vi "updateCommandString.vi"(8 "error in (no error)":errorcluster, 10 "Command U8 Array":u8[](array[numeric]), 11 "MiddlewareSALThisComponent in":refnum<class "MiddlewareSALThisComponent.lvclass">) -> (0 "error out":errorcluster, 2 "Cmd str":string, 3 "MiddlewareSALThisComponent out":refnum<class "MiddlewareSALThisComponent.lvclass">)   [LabVIEW 2016, in "MiddlewareSALThisComponent.lvclass"]
uses:
  MiddlewareSALThisComponent.lvclass
  ComponentTemplateCore/ComponentModel/ComponentModel/Command/Command.lvclass
  SALCommunicatorDL/SALCommunicatorDL.lvclass
  Commands/Start/Start.lvclass
  home/andres/ct_cmpuserevents/CommandThisComponent/CommandThisComponent.lvclass
  home/andres/ct_cmpuserevents/ComponentTemplateCore/ComponentModel/ComponentModel/Command/Command.lvclass
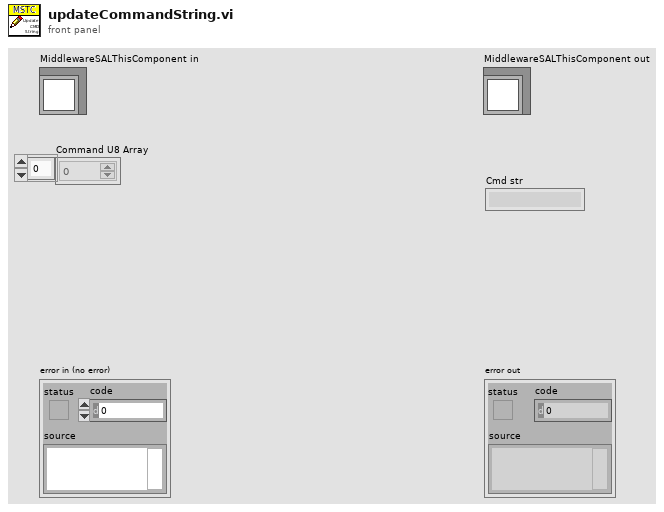
[diagram p1: front panel]
types:
  T1 = enum16{"Command", "Start", "ClearError", "HeartBeat", "Enable", "Disable", "Standby", "Exit", "OnInterrupt", "OnIncomingMessagingError"}
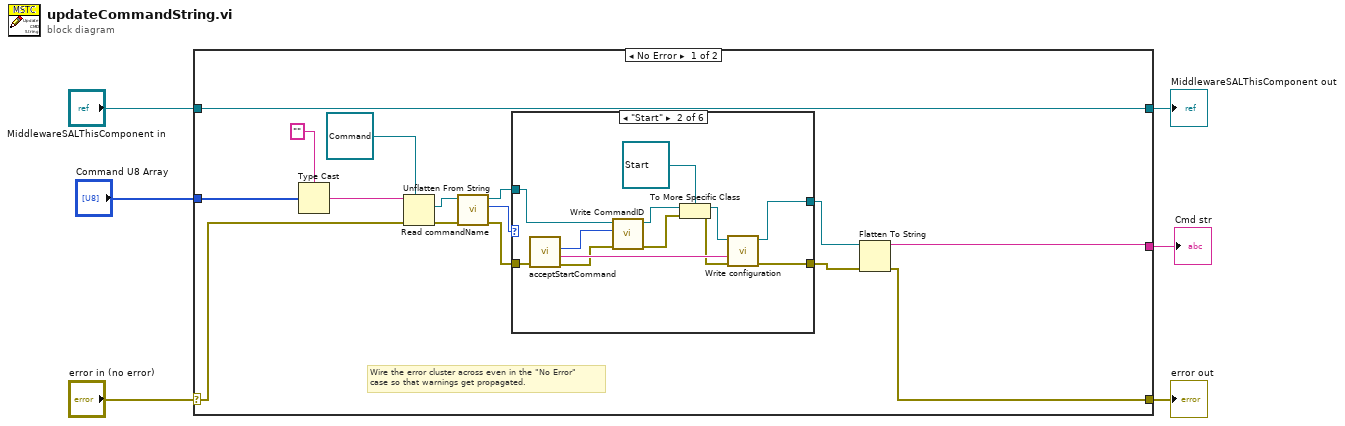
[diagram p0: block diagram]
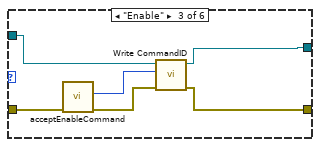
[diagram p3: hidden frame]
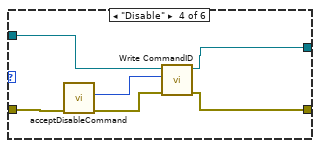
[diagram p4: hidden frame]
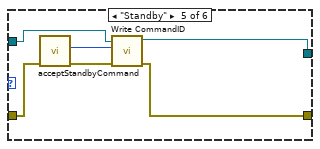
[diagram p5: hidden frame]
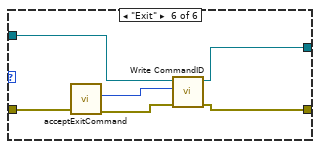
[diagram p6: hidden frame]
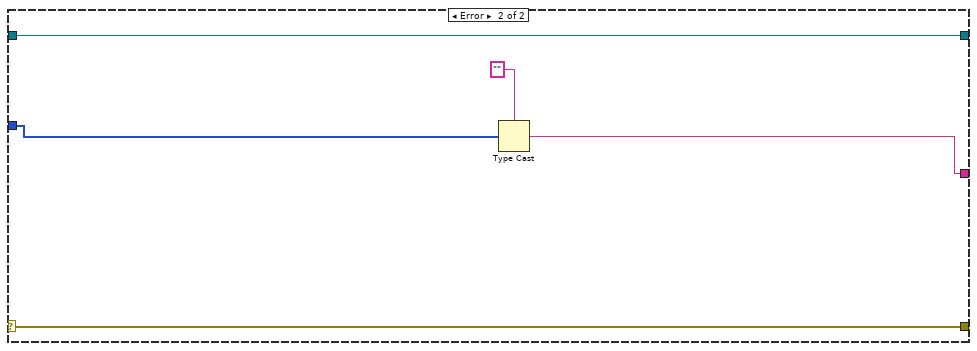
[diagram p7: hidden frame]
diagram:
  n1 = case shown="No Error" "error in (no error)" {
    selector: "error in (no error)" -> [w16 w64]
    tunnel: [w9 w64] -> w5
    tunnel: [w21 w63] -> w3
    tunnel: "MiddlewareSALThisComponent in" -> [w21 w63]
    tunnel: "Command U8 Array" -> [w17 w62]
    tunnel: [w7 w60] -> w1
    frame No Error {
      # "Wire the error cluster across even in the \"No Error\"\ncase so that warnings get propagated."
      n2 = Type Cast(type="", x=w17) -> (*(type *) &x=w18:string)
      n3 = Unflatten From String(type=refnum<class "Command.lvclass"> refnum ("Command.lvclass"), binary string=w18, error in (no error)=w16) -> (value=w14:refnum<class "Command.lvclass">, error out=w15:errorcluster)  [unwired: 2 in, 1 out]
      n4 = call-dynamic "Read commandName.vi"("error in (no error)"=w15, "Command in"=w14) -> ("error out"=w12:errorcluster, "Enum"=w13:T1, "Command out"=w11:refnum<class "Command.lvclass">)  [unwired: 7 in]
      n5 = case shown="\"Start\"" w13 {
        tunnel: w12 -> [w23 w35 w37 w46 w51 w57]
        tunnel: [w23 w30 w40 w42 w49 w54] -> w10
        tunnel: w11 -> [w22 w25 w36 w44 w50 w56]
        tunnel: [w22 w29 w39 w43 w48 w55] -> w8
        frame "Command", Default {
        }
        frame "Start" {
          n6 = call "acceptStartCommand.vi"("error in (no error)"=w35) -> ("error out"=w26:errorcluster, "configuration"=w32:string, "Command ID"=w27:i32)  [unwired: 7 in, 1 out]
          n7 = call-dynamic "Write CommandID.vi"("error in (no error)"=w26, "CommandID"=w27, "Command in"=w25) -> ("error out"=w28:errorcluster, "Command out"=w24:refnum<class "Command.lvclass">)  [unwired: 7 in]
          n8 = To More Specific Class(target class=refnum<class "Start.lvclass"> refnum ("Start in"), reference=w24, error in=w28) -> (specific class reference=w33:refnum<class "Start.lvclass">, error out=w31:errorcluster)
          n9 = call-dynamic "Write configuration.vi"("error in (no error)"=w31, "configuration"=w32, "Start in"=w33) -> ("error out"=w30:errorcluster, "Start out"=w29:refnum<class "Start.lvclass">)  [unwired: 7 in]
        }
        frame "Enable" {
          n10 = call "acceptEnableCommand.vi"("error in (no error)"=w37) -> ("error out"=w41:errorcluster, "Command ID"=w38:i32)  [unwired: 8 in, 1 out]
          n11 = call-dynamic "Write CommandID.vi"("error in (no error)"=w41, "CommandID"=w38, "Command in"=w36) -> ("error out"=w40:errorcluster, "Command out"=w39:refnum<class "Command.lvclass">)  [unwired: 7 in]
        }
        frame "Disable" {
          n12 = call "acceptDisableCommand.vi"("error in (no error)"=w46) -> ("error out"=w47:errorcluster, "Command ID"=w45:i32)  [unwired: 8 in, 1 out]
          n13 = call-dynamic "Write CommandID.vi"("error in (no error)"=w47, "CommandID"=w45, "Command in"=w44) -> ("error out"=w42:errorcluster, "Command out"=w43:refnum<class "Command.lvclass">)  [unwired: 7 in]
        }
        frame "Standby" {
          n14 = call "acceptStandbyCommand.vi"("error in (no error)"=w51) -> ("error out"=w53:errorcluster, "Command ID"=w52:i32)  [unwired: 8 in, 1 out]
          n15 = call-dynamic "Write CommandID.vi"("error in (no error)"=w53, "CommandID"=w52, "Command in"=w50) -> ("error out"=w49:errorcluster, "Command out"=w48:refnum<class "Command.lvclass">)  [unwired: 7 in]
        }
        frame "Exit" {
          n16 = call "acceptExitCommand.vi"("error in (no error)"=w57) -> ("error out"=w59:errorcluster, "Command ID"=w58:i32)  [unwired: 8 in, 1 out]
          n17 = call-dynamic "Write CommandID.vi"("error in (no error)"=w59, "CommandID"=w58, "Command in"=w56) -> ("error out"=w54:errorcluster, "Command out"=w55:refnum<class "Command.lvclass">)  [unwired: 7 in]
        }
      }
      n18 = Flatten To String(anything=w8, error in (no error)=w10) -> (data string=w7:string, error out=w9:errorcluster)  [unwired: 2 in, 1 out]
    }
    frame Error {
      n19 = Type Cast(type="", x=w62) -> (*(type *) &x=w60:string)
    }
  }
  "error out" <- w5
  "MiddlewareSALThisComponent out" <- w3
  "Cmd str" <- w1
